vi "Find Index to Insert at.vi"(8 "Index":i32, 9 "Sections in Target":T1(array[cluster]), 10 "Reference":string, 11 "Target":string) -> (3 "Indices in Ref":i32[](array[numeric]))   [LabVIEW 2020]
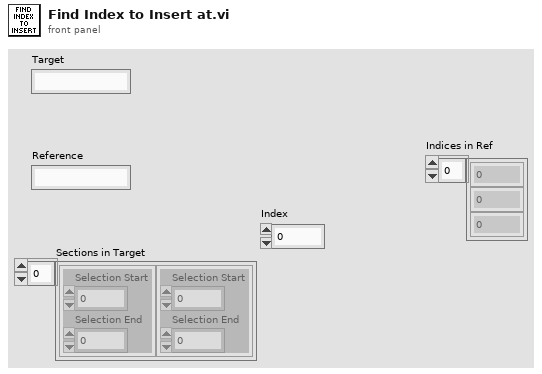
[diagram p1: front panel]
types:
  T1 = cluster{"Selection Start":u32, "Selection End":u32}[]
  T2 = cluster{"Selection Start":u32, "Selection End":u32}
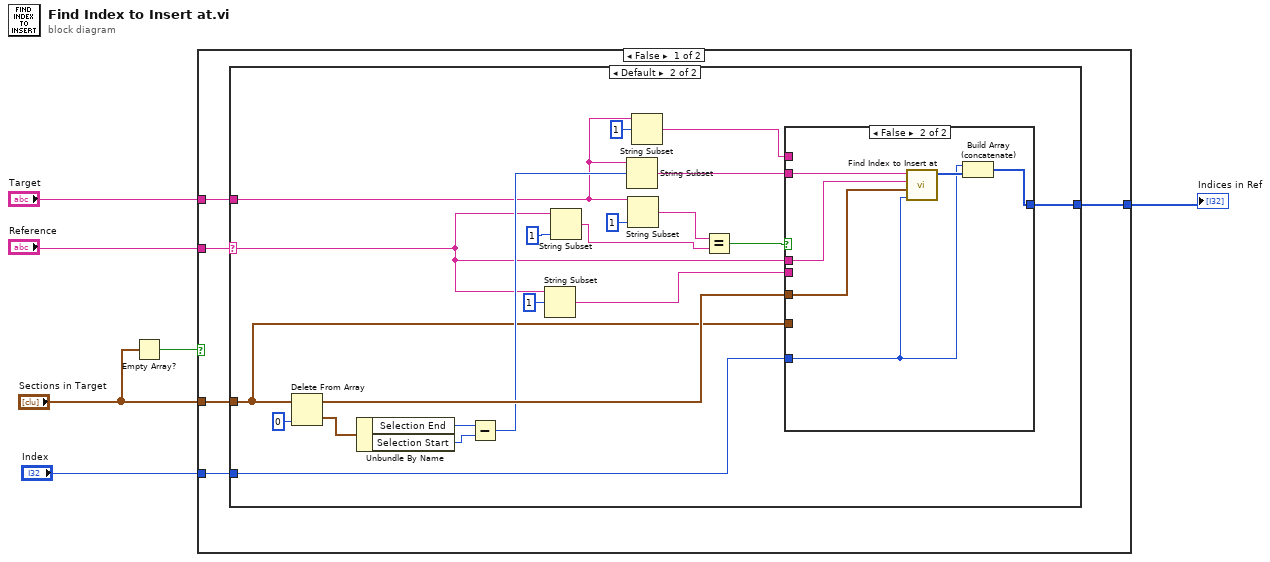
[diagram p0: block diagram]
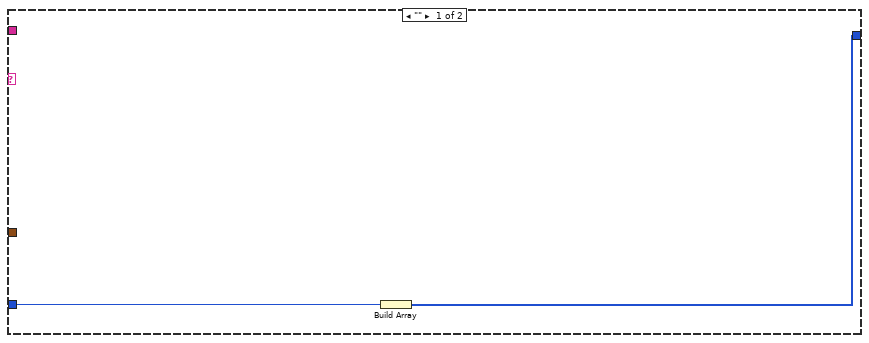
[diagram p2: hidden frame]
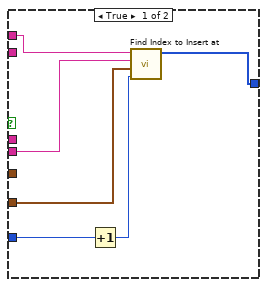
[diagram p3: hidden frame]
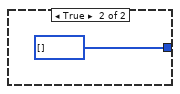
[diagram p4: hidden frame]
diagram:
  n1 = Empty Array?(array="Sections in Target") -> (empty?=w1:bool)
  n2 = case shown="False" w1 {
    tunnel: [w11 i32[] [] ("Indices in Ref")] -> w6
    tunnel: "Reference" -> [w10 _]
    tunnel: "Index" -> [w9 _]
    tunnel: "Target" -> [w8 _]
    tunnel: "Sections in Target" -> [w7 _]
    frame False {
      n3 = case shown="Default" w10 {
        selector: w10 -> [_ w14]
        tunnel: [w12 w32] -> w11
        tunnel: w7 -> [_ w17]
        tunnel: w9 -> [w13 w23]
        tunnel: w8 -> [_ w22]
        frame "" {
          n4 = Build Array(w13) -> (w12:i32[])
        }
        frame Default {
          n5 = Delete From Array(array=w17, index=0) -> (deleted portion=w27:T2, array with subset deleted=w28:T1)  [unwired: 1 in]
          n6 = Unbundle By Name(w27) -> ("Selection End"=w26:u32, "Selection Start"=w25:u32)
          n7 = Subtract(x=w26, y=w25) -> (x-y=w24:u32)
          n8 = String Subset(string=w14, offset (0)=1) -> (substring=w18:string)  [unwired: 1 in]
          n9 = String Subset(string=w14, length (rest)=1 ("offset (0)")) -> (substring=w16:string)  [unwired: 1 in]
          n10 = String Subset(string=w22, offset (0)=w24) -> (substring=w30:string)  [unwired: 1 in]
          n11 = String Subset(string=w22, length (rest)=1 ("length (rest)")) -> (substring=w33:string)  [unwired: 1 in]
          n12 = String Subset(string=w22, offset (0)=1) -> (substring=w20:string)  [unwired: 1 in]
          n13 = Equal?(x=w33, y=w16) -> (x = y?=w31:bool)
          n14 = case shown="False" w31 {
            tunnel: [w40 w42] -> w32
            tunnel: w30 -> [_ w46]
            tunnel: w28 -> [_ w44]
            tunnel: w23 -> [w39 w41]
            tunnel: w20 -> [w37 _]
            tunnel: w18 -> [w36 _]
            tunnel: w17 -> [w35 _]
            tunnel: w14 -> [_ w43]
            frame True {
              n15 = Increment(x=w39) -> (x+1=w38:i32)
              n16 = call "Find Index to Insert at.vi"("Index"=w38, "Sections in Target"=w35, "Reference"=w36, "Target"=w37) -> ("Indices in Ref"=w40:i32[])  [unwired: 7 in]
            }
            frame False {
              n17 = call "Find Index to Insert at.vi"("Index"=w41, "Sections in Target"=w44, "Reference"=w43, "Target"=w46) -> ("Indices in Ref"=w45:i32[])  [unwired: 7 in]
              n18 = Build Array (concatenate)(w41, w45) -> (w42:i32[])
            }
          }
        }
      }
    }
    frame True {
    }
  }
  "Indices in Ref" <- w6
